vi "init_box_2.vi"(0 "Box 2 VISA Name":refnum<visa-resource-name>, 2 "Trap Delay Array":dbl[](array[numeric]), 7 "Controls Cluster":T1, 11 "error in (no error)":errorcluster, 13 "Laser In Use":string(combo)) -> (4 "Box 2 VISA Name Out":refnum<visa-resource-name>, 15 "Error out":errorcluster)   [LabVIEW 2023]
uses:
  <instrlib>/Quantum Composers 9000 Series/Public/Configure/Configure Chan Mode (Normal).vi
  <instrlib>/Quantum Composers 9000 Series/Quantum Composers 9000 Series.lvlib
  <instrlib>/Quantum Composers 9000 Series/Public/Action-Status/Query Sys (To) Parameters (Input).vi
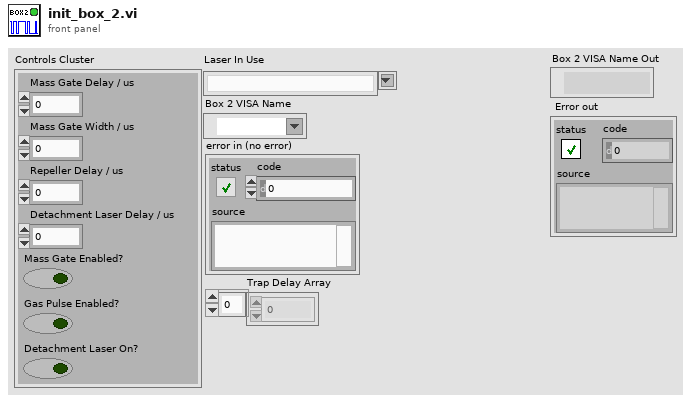
[diagram p1: front panel]
types:
  T1 = cluster{"Mass Gate Delay / us":dbl, "Mass Gate Width / us":dbl, "Repeller Delay / us":dbl, "Detachment Laser Delay / us":dbl, "Mass Gate Enabled?":bool, "Gas Pulse Enabled?":bool, "Detachment Laser On?":bool}
  T2 = enum16{"Disabled", "Triggered", "Gated", "Triggered & Gated"}
  T3 = enum16{"Disabled", "Pulse Inhibit", "Output Inhibit"}
  T4 = cluster{"Sys Ext Mode":enum16{"Disabled", "Triggered", "Gated", "Triggered & Gated"}, "Trig Level":dbl, "Trig Edge":bool, "Gate Logic":bool, "Gate Level":dbl, "Gate Mode":enum16{"Disabled", "Pulse Inhibit", "Output Inhibit", "Channel"}}
  T5 = enum16{"Disabled", "Pulse Inhibit", "Output Inhibit", "Channel"}
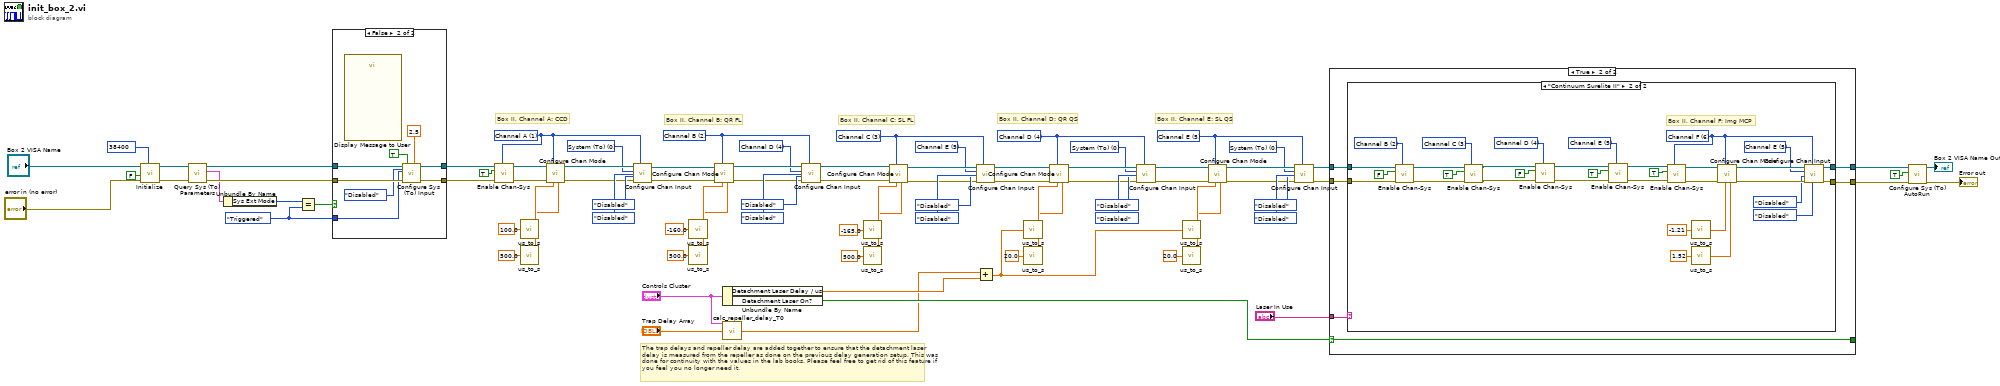
[diagram p0: block diagram]
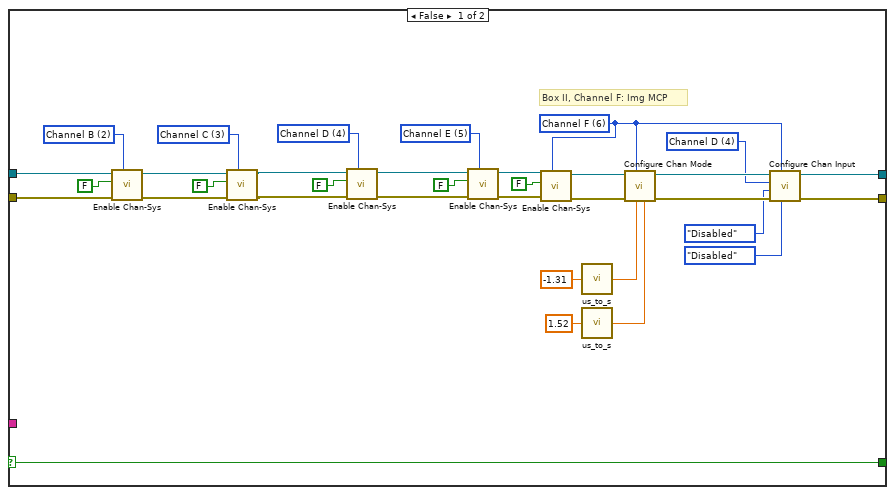
[diagram p3: hidden frame]
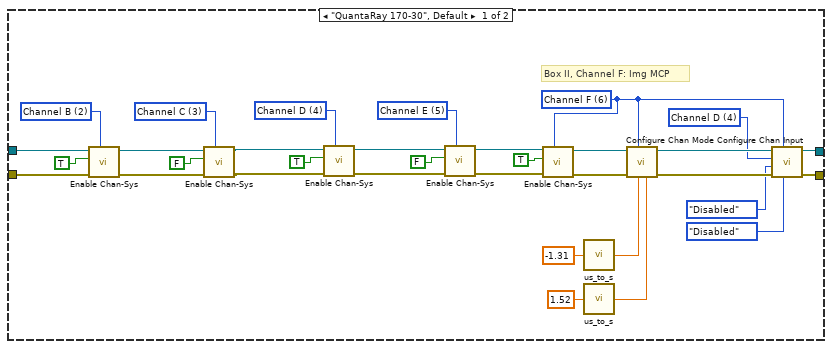
[diagram p4: hidden frame]
diagram:
  w2 = T2."Triggered" ("Sys Ext Mode")
  w10 = u32 38400 items=["4800"=4600, "9600"=9600, "19200"=19200, "38400"=38400, "57600"=57600, "115200"=115200] ("Baud Rate (9600)")
  w28 = 0 items=["System (To)", "Channel A", "Channel B", "Channel C", "Channel D", "Channel E", "Channel F", "Channel G", "Channel H"] ("Sync Source (0:To)")
  w27 = 5 items=["Channel A"=1, "Channel B"=2, "Channel C"=3, "Channel D"=4, "Channel E"=5, "Channel F"=6, "Channel G"=7, "Channel H"=8] ("Channel (1:Chan A)")
  w39 = 0 items=["System (To)", "Channel A", "Channel B", "Channel C", "Channel D", "Channel E", "Channel F", "Channel G", "Channel H"] ("Sync Source (0:To)")
  w38 = 4 items=["Channel A"=1, "Channel B"=2, "Channel C"=3, "Channel D"=4, "Channel E"=5, "Channel F"=6, "Channel G"=7, "Channel H"=8] ("Channel (1:Chan A)")
  w51 = 5 items=["System (To)", "Channel A", "Channel B", "Channel C", "Channel D", "Channel E", "Channel F", "Channel G", "Channel H"] ("Sync Source (0:To)")
  w49 = 3 items=["Channel A"=1, "Channel B"=2, "Channel C"=3, "Channel D"=4, "Channel E"=5, "Channel F"=6, "Channel G"=7, "Channel H"=8] ("Channel (1:Chan A)")
  w63 = 4 items=["System (To)", "Channel A", "Channel B", "Channel C", "Channel D", "Channel E", "Channel F", "Channel G", "Channel H"] ("Sync Source (0:To)")
  w61 = 2 items=["Channel A"=1, "Channel B"=2, "Channel C"=3, "Channel D"=4, "Channel E"=5, "Channel F"=6, "Channel G"=7, "Channel H"=8] ("Channel (1:Chan A)")
  w79 = 0 items=["System (To)", "Channel A", "Channel B", "Channel C", "Channel D", "Channel E", "Channel F", "Channel G", "Channel H"] ("Sync Source (0:To)")
  w75 = 1 items=["Channel A"=1, "Channel B"=2, "Channel C"=3, "Channel D"=4, "Channel E"=5, "Channel F"=6, "Channel G"=7, "Channel H"=8] ("Channel (1:Chan A)")
  # "The trap delays and repeller delay are added together to ensure that the detachment laser delay is measured from the repeller as done on the previous delay generation setup. This was done for continuity with the values in the lab books. Please feel free to get rid of this feature if you feel you no longer need it."
  # "Box II, Channel E: SL QS"
  # "Box II, Channel D: QR QS"
  # "Box II, Channel C: SL FL"
  # "Box II, Channel B: QR FL"
  # "Box II, Channel A: CCD"
  n1 = call <instrlib>:"Initialize.vi"("Baud Rate (9600)"=w10, "error in (no error)"="error in (no error)", "Reset? (T: Yes)"=FALSE, "VISA resource name"="Box 2 VISA Name") -> ("error out"=w7:errorcluster, "VISA resource name out"=w8:refnum<visa-resource-name>)  [unwired: 6 in]
  n2 = call-poly <instrlib>:"Query Sys (To) Parameters.vi"("error in (no error)"=w7, "VISA resource name"=w8) -> ("error out"=w5:errorcluster, "Input Parameters"=w4:T4, "VISA resource name out"=w6:refnum<visa-resource-name>)  [unwired: 7 in]
  n3 = Unbundle By Name(w4) -> ("Sys Ext Mode"=w3:T2)
  n4 = Equal?(x=w3, y=w2) -> (x = y?=w1:bool)
  n5 = case shown="False" w1 {
    tunnel: w6 -> [w89 w97]
    tunnel: w5 -> [w88 w96]
    tunnel: [w89 w93] -> w73
    tunnel: [w88 w92] -> w72
    tunnel: w2 -> [_ w90]
    frame True {
    }
    frame False {
      n6 = call "Display Message to User"() -> ()  [unwired: 10 in, 2 out]
      n7 = call <instrlib>:"Configure Sys (To) Input.vi"("Sys Trig Lev (2.5)"=2.5, "Sys Gate Mode"=T5."Disabled", "Sys Trig Edge (T: Rising)"=TRUE, "error in (no error)"=w96, "Sys Ext Mode"=w90, "VISA resource name"=w97) -> ("error out"=w92:errorcluster, "VISA resource name out"=w93:refnum<visa-resource-name>)  [unwired: 4 in]
    }
  }
  n8 = call <instrlib>:"Enable Chan-Sys.vi"("Channel (1:Chan A)"=w75, "error in (no error)"=w72, "State (T:Enabled)"=TRUE, "VISA resource name"=w73) -> ("error out"=w76:errorcluster, "VISA resource name out"=w77:refnum<visa-resource-name>)  [unwired: 6 in]
  n9 = call "us_to_s.vi"("Time / us"=100.0) -> ("Time / s"=w83:dbl)
  n10 = call "us_to_s.vi"("Time / us"=500.0) -> ("Time / s"=w82:dbl)
  n11 = call-poly <instrlib>:"Configure Chan Mode.vi"("Width (10 msec)"=w82, "Delay (10 msec)"=w83, "Channel (1:Chan A)"=w75, "error in (no error)"=w76, "VISA resource name"=w77) -> ("error out"=w84:errorcluster, "VISA resource name out"=w85:refnum<visa-resource-name>)  [unwired: 5 in]
  n12 = call <instrlib>:"Configure Chan Input.vi"("Gate Mode (0:Disabled)"=T3."Disabled", "Channel (1:Chan A)"=w75, "error in (no error)"=w84, "Gate Logic (0:Disabled)"=enum16{"Disabled", "Low", "High"}."Disabled", "Sync Source (0:To)"=w79, "VISA resource name"=w85) -> ("error out"=w59:errorcluster, "VISA resource name out"=w60:refnum<visa-resource-name>)  [unwired: 4 in]
  n13 = call "us_to_s.vi"("Time / us"=-160.0) -> ("Time / s"=w66:dbl)
  n14 = call "us_to_s.vi"("Time / us"=500.0) -> ("Time / s"=w65:dbl)
  n15 = call-poly <instrlib>:"Configure Chan Mode.vi"("Width (10 msec)"=w65, "Delay (10 msec)"=w66, "Channel (1:Chan A)"=w61, "error in (no error)"=w59, "VISA resource name"=w60) -> ("error out"=w67:errorcluster, "VISA resource name out"=w68:refnum<visa-resource-name>)  [unwired: 5 in]
  n16 = Unbundle By Name("Controls Cluster") -> ("Detachment Laser Delay / us"=w15:dbl, "Detachment Laser On?"=w19:bool)
  n17 = call "calc_repeller_delay_T0.vi"("Variable Values Out"="Controls Cluster", "Trap Delay Array"="Trap Delay Array") -> ("Total Repeller Delay / us"=w12:dbl)  [unwired: 13 in]
  n18 = call <instrlib>:"Configure Chan Input.vi"("Gate Mode (0:Disabled)"=T3."Disabled", "Channel (1:Chan A)"=w61, "error in (no error)"=w67, "Gate Logic (0:Disabled)"=enum16{"Disabled", "Low", "High"}."Disabled", "Sync Source (0:To)"=w63, "VISA resource name"=w68) -> ("error out"=w47:errorcluster, "VISA resource name out"=w48:refnum<visa-resource-name>)  [unwired: 4 in]
  n19 = call "us_to_s.vi"("Time / us"=-165.0) -> ("Time / s"=w54:dbl)
  n20 = call "us_to_s.vi"("Time / us"=500.0) -> ("Time / s"=w53:dbl)
  n21 = call-poly <instrlib>:"Configure Chan Mode.vi"("Width (10 msec)"=w53, "Delay (10 msec)"=w54, "Channel (1:Chan A)"=w49, "error in (no error)"=w47, "VISA resource name"=w48) -> ("error out"=w55:errorcluster, "VISA resource name out"=w56:refnum<visa-resource-name>)  [unwired: 5 in]
  n22 = call <instrlib>:"Configure Chan Input.vi"("Gate Mode (0:Disabled)"=T3."Disabled", "Channel (1:Chan A)"=w49, "error in (no error)"=w55, "Gate Logic (0:Disabled)"=enum16{"Disabled", "Low", "High"}."Disabled", "Sync Source (0:To)"=w51, "VISA resource name"=w56) -> ("error out"=w36:errorcluster, "VISA resource name out"=w37:refnum<visa-resource-name>)  [unwired: 4 in]
  n23 = Add(x=w12, y=w15) -> (x+y=w11:dbl)
  n24 = call "us_to_s.vi"("Time / us"=w11) -> ("Time / s"=w42:dbl)
  n25 = call "us_to_s.vi"("Time / us"=20.0) -> ("Time / s"=w41:dbl)
  n26 = call-poly <instrlib>:"Configure Chan Mode.vi"("Width (10 msec)"=w41, "Delay (10 msec)"=w42, "Channel (1:Chan A)"=w38, "error in (no error)"=w36, "VISA resource name"=w37) -> ("error out"=w43:errorcluster, "VISA resource name out"=w44:refnum<visa-resource-name>)  [unwired: 5 in]
  n27 = call <instrlib>:"Configure Chan Input.vi"("Gate Mode (0:Disabled)"=T3."Disabled", "Channel (1:Chan A)"=w38, "error in (no error)"=w43, "Gate Logic (0:Disabled)"=enum16{"Disabled", "Low", "High"}."Disabled", "Sync Source (0:To)"=w39, "VISA resource name"=w44) -> ("error out"=w25:errorcluster, "VISA resource name out"=w26:refnum<visa-resource-name>)  [unwired: 4 in]
  n28 = call "us_to_s.vi"("Time / us"=w11) -> ("Time / s"=w31:dbl)
  n29 = call "us_to_s.vi"("Time / us"=20.0) -> ("Time / s"=w30:dbl)
  n30 = call-poly <instrlib>:"Configure Chan Mode.vi"("Width (10 msec)"=w30, "Delay (10 msec)"=w31, "Channel (1:Chan A)"=w27, "error in (no error)"=w25, "VISA resource name"=w26) -> ("error out"=w32:errorcluster, "VISA resource name out"=w33:refnum<visa-resource-name>)  [unwired: 5 in]
  n31 = call <instrlib>:"Configure Chan Input.vi"("Gate Mode (0:Disabled)"=T3."Disabled", "Channel (1:Chan A)"=w27, "error in (no error)"=w32, "Gate Logic (0:Disabled)"=enum16{"Disabled", "Low", "High"}."Disabled", "Sync Source (0:To)"=w28, "VISA resource name"=w33) -> ("error out"=w23:errorcluster, "VISA resource name out"=w24:refnum<visa-resource-name>)  [unwired: 4 in]
  n32 = case shown="True" w19 {
    selector: w19 -> [w98 w132]
    tunnel: "Laser In Use" -> [_ w137]
    tunnel: w24 -> [w129 w136]
    tunnel: w23 -> [w128 w135]
    tunnel: [w102 w134] -> w22
    tunnel: [w101 w133] -> w21
    tunnel: [w98 w132] -> _
    frame False {
      w107 = 4 items=["System (To)", "Channel A", "Channel B", "Channel C", "Channel D", "Channel E", "Channel F", "Channel G", "Channel H"] ("Sync Source (0:To)")
      w104 = 6 items=["Channel A"=1, "Channel B"=2, "Channel C"=3, "Channel D"=4, "Channel E"=5, "Channel F"=6, "Channel G"=7, "Channel H"=8] ("Channel (1:Chan A)")
      w119 = 5 items=["System (To)", "Channel A", "Channel B", "Channel C", "Channel D", "Channel E", "Channel F", "Channel G", "Channel H"] ("Channel (1:Chan A)")
      w123 = 4 items=["System (To)", "Channel A", "Channel B", "Channel C", "Channel D", "Channel E", "Channel F", "Channel G", "Channel H"] ("Channel (1:Chan A)")
      w127 = 3 items=["System (To)", "Channel A", "Channel B", "Channel C", "Channel D", "Channel E", "Channel F", "Channel G", "Channel H"] ("Channel (1:Chan A)")
      w131 = 2 items=["System (To)", "Channel A", "Channel B", "Channel C", "Channel D", "Channel E", "Channel F", "Channel G", "Channel H"] ("Channel (1:Chan A)")
      # "Box II, Channel F: Img MCP"
      n33 = call <instrlib>:"Enable Chan-Sys.vi"("Channel (1:Chan A)"=w131, "error in (no error)"=w128, "State (T:Enabled)"=FALSE, "VISA resource name"=w129) -> ("error out"=w124:errorcluster, "VISA resource name out"=w125:refnum<visa-resource-name>)  [unwired: 6 in]
      n34 = call <instrlib>:"Enable Chan-Sys.vi"("Channel (1:Chan A)"=w127, "error in (no error)"=w124, "State (T:Enabled)"=FALSE, "VISA resource name"=w125) -> ("error out"=w120:errorcluster, "VISA resource name out"=w121:refnum<visa-resource-name>)  [unwired: 6 in]
      n35 = call <instrlib>:"Enable Chan-Sys.vi"("Channel (1:Chan A)"=w123, "error in (no error)"=w120, "State (T:Enabled)"=FALSE, "VISA resource name"=w121) -> ("error out"=w116:errorcluster, "VISA resource name out"=w117:refnum<visa-resource-name>)  [unwired: 6 in]
      n36 = call <instrlib>:"Enable Chan-Sys.vi"("Channel (1:Chan A)"=w119, "error in (no error)"=w116, "State (T:Enabled)"=FALSE, "VISA resource name"=w117) -> ("error out"=w99:errorcluster, "VISA resource name out"=w100:refnum<visa-resource-name>)  [unwired: 6 in]
      n37 = call <instrlib>:"Enable Chan-Sys.vi"("Channel (1:Chan A)"=w104, "error in (no error)"=w99, "State (T:Enabled)"=FALSE, "VISA resource name"=w100) -> ("error out"=w105:errorcluster, "VISA resource name out"=w106:refnum<visa-resource-name>)  [unwired: 6 in]
      n38 = call "us_to_s.vi"("Time / us"=-1.31) -> ("Time / s"=w114:dbl)
      n39 = call "us_to_s.vi"("Time / us"=1.52) -> ("Time / s"=w115:dbl)
      n40 = call-poly <instrlib>:"Configure Chan Mode.vi"("Width (10 msec)"=w115, "Delay (10 msec)"=w114, "Channel (1:Chan A)"=w104, "error in (no error)"=w105, "VISA resource name"=w106) -> ("error out"=w113:errorcluster, "VISA resource name out"=w112:refnum<visa-resource-name>)  [unwired: 5 in]
      n41 = call <instrlib>:"Configure Chan Input.vi"("Gate Mode (0:Disabled)"=T3."Disabled", "Channel (1:Chan A)"=w104, "error in (no error)"=w113, "Gate Logic (0:Disabled)"=enum16{"Disabled", "Low", "High"}."Disabled", "Sync Source (0:To)"=w107, "VISA resource name"=w112) -> ("error out"=w101:errorcluster, "VISA resource name out"=w102:refnum<visa-resource-name>)  [unwired: 4 in]
    }
    frame True {
      n42 = case shown="\"Continuum Surelite II\"" w137 {
        tunnel: w136 -> [w143 w176]
        tunnel: w135 -> [w142 w175]
        tunnel: [w141 w174] -> w134
        tunnel: [w140 w173] -> w133
        frame "QuantaRay 170-30", Default {
          w148 = 4 items=["System (To)", "Channel A", "Channel B", "Channel C", "Channel D", "Channel E", "Channel F", "Channel G", "Channel H"] ("Sync Source (0:To)")
          w145 = 6 items=["Channel A"=1, "Channel B"=2, "Channel C"=3, "Channel D"=4, "Channel E"=5, "Channel F"=6, "Channel G"=7, "Channel H"=8] ("Channel (1:Chan A)")
          w160 = 5 items=["System (To)", "Channel A", "Channel B", "Channel C", "Channel D", "Channel E", "Channel F", "Channel G", "Channel H"] ("Channel (1:Chan A)")
          w164 = 4 items=["System (To)", "Channel A", "Channel B", "Channel C", "Channel D", "Channel E", "Channel F", "Channel G", "Channel H"] ("Channel (1:Chan A)")
          w168 = 3 items=["System (To)", "Channel A", "Channel B", "Channel C", "Channel D", "Channel E", "Channel F", "Channel G", "Channel H"] ("Channel (1:Chan A)")
          w170 = 2 items=["System (To)", "Channel A", "Channel B", "Channel C", "Channel D", "Channel E", "Channel F", "Channel G", "Channel H"] ("Channel (1:Chan A)")
          # "Box II, Channel F: Img MCP"
          n43 = call <instrlib>:"Enable Chan-Sys.vi"("Channel (1:Chan A)"=w170, "error in (no error)"=w142, "State (T:Enabled)"=TRUE, "VISA resource name"=w143) -> ("error out"=w165:errorcluster, "VISA resource name out"=w166:refnum<visa-resource-name>)  [unwired: 6 in]
          n44 = call <instrlib>:"Enable Chan-Sys.vi"("Channel (1:Chan A)"=w168, "error in (no error)"=w165, "State (T:Enabled)"=FALSE, "VISA resource name"=w166) -> ("error out"=w161:errorcluster, "VISA resource name out"=w162:refnum<visa-resource-name>)  [unwired: 6 in]
          n45 = call <instrlib>:"Enable Chan-Sys.vi"("Channel (1:Chan A)"=w164, "error in (no error)"=w161, "State (T:Enabled)"=TRUE, "VISA resource name"=w162) -> ("error out"=w157:errorcluster, "VISA resource name out"=w158:refnum<visa-resource-name>)  [unwired: 6 in]
          n46 = call <instrlib>:"Enable Chan-Sys.vi"("Channel (1:Chan A)"=w160, "error in (no error)"=w157, "State (T:Enabled)"=FALSE, "VISA resource name"=w158) -> ("error out"=w138:errorcluster, "VISA resource name out"=w139:refnum<visa-resource-name>)  [unwired: 6 in]
          n47 = call <instrlib>:"Enable Chan-Sys.vi"("Channel (1:Chan A)"=w145, "error in (no error)"=w138, "State (T:Enabled)"=TRUE, "VISA resource name"=w139) -> ("error out"=w146:errorcluster, "VISA resource name out"=w147:refnum<visa-resource-name>)  [unwired: 6 in]
          n48 = call "us_to_s.vi"("Time / us"=-1.31) -> ("Time / s"=w155:dbl)
          n49 = call "us_to_s.vi"("Time / us"=1.52) -> ("Time / s"=w156:dbl)
          n50 = call-poly <instrlib>:"Configure Chan Mode.vi"("Width (10 msec)"=w156, "Delay (10 msec)"=w155, "Channel (1:Chan A)"=w145, "error in (no error)"=w146, "VISA resource name"=w147) -> ("error out"=w154:errorcluster, "VISA resource name out"=w153:refnum<visa-resource-name>)  [unwired: 5 in]
          n51 = call <instrlib>:"Configure Chan Input.vi"("Gate Mode (0:Disabled)"=T3."Disabled", "Channel (1:Chan A)"=w145, "error in (no error)"=w154, "Gate Logic (0:Disabled)"=enum16{"Disabled", "Low", "High"}."Disabled", "Sync Source (0:To)"=w148, "VISA resource name"=w153) -> ("error out"=w140:errorcluster, "VISA resource name out"=w141:refnum<visa-resource-name>)  [unwired: 4 in]
        }
        frame "Continuum Surelite II" {
          w181 = 5 items=["System (To)", "Channel A", "Channel B", "Channel C", "Channel D", "Channel E", "Channel F", "Channel G", "Channel H"] ("Sync Source (0:To)")
          w178 = 6 items=["Channel A"=1, "Channel B"=2, "Channel C"=3, "Channel D"=4, "Channel E"=5, "Channel F"=6, "Channel G"=7, "Channel H"=8] ("Channel (1:Chan A)")
          w193 = 5 items=["System (To)", "Channel A", "Channel B", "Channel C", "Channel D", "Channel E", "Channel F", "Channel G", "Channel H"] ("Channel (1:Chan A)")
          w197 = 4 items=["System (To)", "Channel A", "Channel B", "Channel C", "Channel D", "Channel E", "Channel F", "Channel G", "Channel H"] ("Channel (1:Chan A)")
          w201 = 3 items=["System (To)", "Channel A", "Channel B", "Channel C", "Channel D", "Channel E", "Channel F", "Channel G", "Channel H"] ("Channel (1:Chan A)")
          w203 = 2 items=["System (To)", "Channel A", "Channel B", "Channel C", "Channel D", "Channel E", "Channel F", "Channel G", "Channel H"] ("Channel (1:Chan A)")
          # "Box II, Channel F: Img MCP"
          n52 = call <instrlib>:"Enable Chan-Sys.vi"("Channel (1:Chan A)"=w203, "error in (no error)"=w175, "State (T:Enabled)"=FALSE, "VISA resource name"=w176) -> ("error out"=w198:errorcluster, "VISA resource name out"=w199:refnum<visa-resource-name>)  [unwired: 6 in]
          n53 = call <instrlib>:"Enable Chan-Sys.vi"("Channel (1:Chan A)"=w201, "error in (no error)"=w198, "State (T:Enabled)"=TRUE, "VISA resource name"=w199) -> ("error out"=w194:errorcluster, "VISA resource name out"=w195:refnum<visa-resource-name>)  [unwired: 6 in]
          n54 = call <instrlib>:"Enable Chan-Sys.vi"("Channel (1:Chan A)"=w197, "error in (no error)"=w194, "State (T:Enabled)"=FALSE, "VISA resource name"=w195) -> ("error out"=w190:errorcluster, "VISA resource name out"=w191:refnum<visa-resource-name>)  [unwired: 6 in]
          n55 = call <instrlib>:"Enable Chan-Sys.vi"("Channel (1:Chan A)"=w193, "error in (no error)"=w190, "State (T:Enabled)"=TRUE, "VISA resource name"=w191) -> ("error out"=w171:errorcluster, "VISA resource name out"=w172:refnum<visa-resource-name>)  [unwired: 6 in]
          n56 = call <instrlib>:"Enable Chan-Sys.vi"("Channel (1:Chan A)"=w178, "error in (no error)"=w171, "State (T:Enabled)"=TRUE, "VISA resource name"=w172) -> ("error out"=w179:errorcluster, "VISA resource name out"=w180:refnum<visa-resource-name>)  [unwired: 6 in]
          n57 = call "us_to_s.vi"("Time / us"=-1.21) -> ("Time / s"=w188:dbl)
          n58 = call "us_to_s.vi"("Time / us"=1.52) -> ("Time / s"=w189:dbl)
          n59 = call-poly <instrlib>:"Configure Chan Mode.vi"("Width (10 msec)"=w189, "Delay (10 msec)"=w188, "Channel (1:Chan A)"=w178, "error in (no error)"=w179, "VISA resource name"=w180) -> ("error out"=w187:errorcluster, "VISA resource name out"=w186:refnum<visa-resource-name>)  [unwired: 5 in]
          n60 = call <instrlib>:"Configure Chan Input.vi"("Gate Mode (0:Disabled)"=T3."Disabled", "Channel (1:Chan A)"=w178, "error in (no error)"=w187, "Gate Logic (0:Disabled)"=enum16{"Disabled", "Low", "High"}."Disabled", "Sync Source (0:To)"=w181, "VISA resource name"=w186) -> ("error out"=w173:errorcluster, "VISA resource name out"=w174:refnum<visa-resource-name>)  [unwired: 4 in]
        }
      }
    }
  }
  n61 = call <instrlib>:"Configure Sys (To) AutoRun.vi"("error in (no error)"=w21, "AutoRun (F:Disabled)"=TRUE, "VISA resource name"=w22) -> ("error out"=→"Error out":errorcluster, "VISA resource name out"=→"Box 2 VISA Name Out":refnum<visa-resource-name>)  [unwired: 7 in]
